vi "main.vi"() -> ()   [LabVIEW 2012]
panel:
  out "Modulo":dbl
  in  "stop":bool
  in  "OK Button":bool
  out "Altura (deg)":dbl(knob) scale=-90.0..90.0
  out "Azimute (deg)":dbl(knob) scale=0.0..360.0
  in  "Latitude Local (deg)":dbl(knob) scale=-90.0..90.0
  in  "AH (h)":dbl(knob) scale=-6.0..6.0
  in  "DEC (deg)":dbl(knob) scale=-50.0..30.0
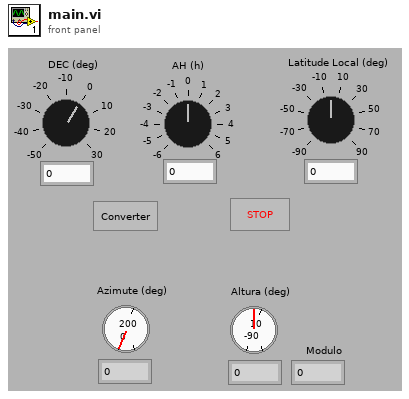
[diagram p1: front panel]
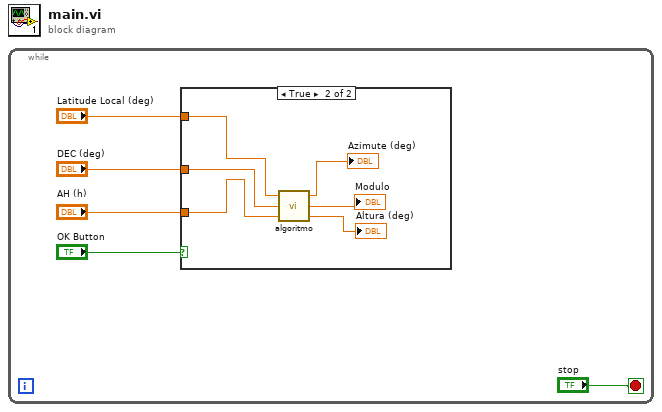
[diagram p0: block diagram]
diagram:
  n1 = while {
    stop <- "stop" stop-if-true
    n2 = case shown="True" "OK Button" {
      tunnel: "Latitude Local (deg)" -> [_ w11]
      tunnel: "AH (h)" -> [_ w9]
      tunnel: "DEC (deg)" -> [_ w10]
      frame False {
      }
      frame True {
        n3 = call "algoritmo.vi"("AH"=w9, "DEC"=w10, "Latitude Local"=w11) -> ("Altura"=→"Altura (deg)":dbl, "Módulo da Altura"=→"Modulo":dbl, "Azimute"=→"Azimute (deg)":dbl)
      }
    }
  }
